vi "PH_AxisGUI_BaseClass.set GUI Refs.vi"(0 "i ref in":refnum<vi>, 2 "Class":string, 3 "Axis GUI Base Class Refs":T1[](array[typedef]), 5 "error in":errorcluster) -> (14 "i ref out":refnum<vi>, 19 "error out":errorcluster)   [LabVIEW 2014, in "PH_AxisGUI_BaseClass.lvlib"]
doc: "This VI is forseen to set the GUI element references; it shall be used especially within child classes."
uses:
  PH_AxisGUI_BaseClass.lvlib
  PH_AxisGUI_BaseClass.Axis GUI Refs.ctl
  PH_Stepmotor_BaseClass/PH_Stepmotor_BaseClass.Axis Address.ctl
  PH_Stepmotor_BaseClass/PH_Stepmotor_BaseClass.Axis Settings.ctl
  PH_Stepmotor_BaseClass/PH_Stepmotor_BaseClass.Motor Type.ctl
  PH_Stepmotor_BaseClass/PH_Stepmotor_BaseClass.Axis Activity.ctl
  PH_Stepmotor_BaseClass/PH_Stepmotor_BaseClass.lvlib
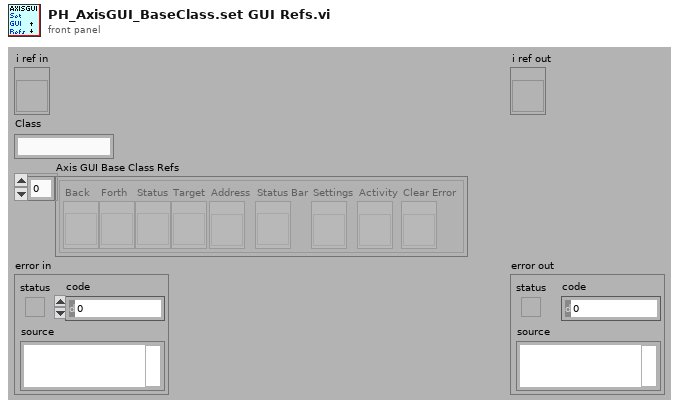
[diagram p1: front panel]
types:
  T1 = typedef "PH_AxisGUI_BaseClass.lvlib/PH_AxisGUI_BaseClass.Axis GUI Refs.ctl" = cluster{"Back":refnum<vi>, "Forth":refnum<vi>, "Status":refnum<vi>, "Target":refnum<vi>, "Address":refnum<vi>, "Status Bar":refnum<vi>, "Settings":refnum<vi>, "Activity":refnum<vi>, "Clear Error":refnum<vi>}
  T2 = typedef "PH_AxisGUI_BaseClass.lvlib/PH_AxisGUI_BaseClass.i attribute.ctl" = cluster{"Axes":T3[]}
  T3 = typedef "PH_AxisGUI_BaseClass.lvlib/PH_AxisGUI_BaseClass.Axis Attributes.ctl" = cluster{"Axis GUI Refs":T1, "Address":T4, "Name":string, "Label \"Back\"":string, "Labell \"Forth\"":string, "Moving?":bool}
  T4 = typedef "PH_Stepmotor_BaseClass.lvlib/PH_Stepmotor_BaseClass.Axis Address.ctl" = cluster{"Instance":string, "Motor Nr":i32}
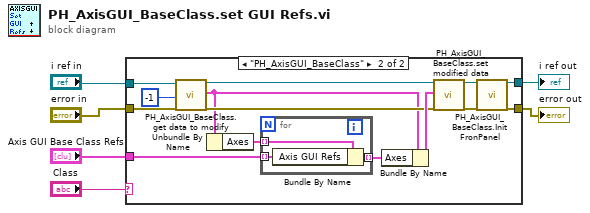
[diagram p0: block diagram]
diagram:
  n1 = case shown="\"PH_AxisGUI_BaseClass\"" "Class" {
    tunnel: "error in" -> [w7 w21]
    tunnel: "i ref in" -> [w8 w20]
    tunnel: "Axis GUI Base Class Refs" -> [_ w15]
    tunnel: [w8 w11] -> w3
    tunnel: [w7 w10] -> w2
    frame Default {
    }
    frame "PH_AxisGUI_BaseClass" {
      n2 = call "PH_AxisGUI_BaseClass.get data to modify.vi"("i ref in"=w20, "ms timeout (10000)"=-1, "error in (no error)"=w21) -> ("i ref out"=w17:refnum<vi>, "i attribute"=w16:T2, "error out"=w18:errorcluster)  [unwired: 13 in, 1 out]
      n3 = Unbundle By Name(w16) -> ("Axes"=w14:T3[])
      n4 = for {
        tunnel: w14 -> [w25] mode=indexing
        tunnel: [w24] -> w9 mode=indexing
        tunnel: w15 -> [w23] mode=indexing
        n5 = Bundle By Name(cluster=w25, "Axis GUI Refs"=w23) -> (w24:T3)
      }
      n6 = Bundle By Name(cluster=w16, "Axes"=w9) -> (w22:T2)
      n7 = call "PH_AxisGUI_BaseClass.set modified data.vi"("i ref in"=w17, "i attribute"=w22, "error in (no error)"=w18) -> ("i ref out"=w13:refnum<vi>, "error out"=w12:errorcluster)  [unwired: 15 in]
      n8 = call "PH_AxisGUI_BaseClass.Init FronPanel.vi"("i ref in"=w13, "error in"=w12) -> ("i ref out"=w11:refnum<vi>, "error out"=w10:errorcluster)  [unwired: 16 in]
    }
  }
  "error out" <- w2
  "i ref out" <- w3
